vi "JSONRPC-BuildResponse.vi"(7 "ID":string="{\\\"jsonrpc\\\":\"2.0\",\\\"result\\\":%s,\\\"id\\\":%s}", 8 "error in":errorcluster, 11 "Result":string="{\\\"jsonrpc\\\":\"2.0\",\\\"result\\\":%s,\\\"id\\\":%s}") -> (0 "error out":errorcluster, 3 "JSONRPC Response":string)   [LabVIEW 2013]
doc: "Build a JSONRPC 2.0 response with <b>result</b>, or a JSONRPC 2.0 error response if <b>error in</b> contains an error. The response is bound to <b>ID</b>."
panel:
  # "BuildResponse"
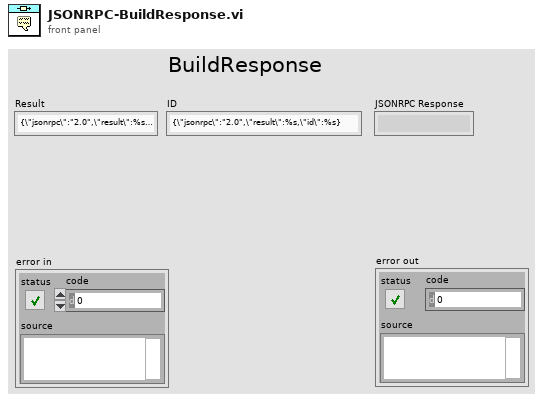
[diagram p1: front panel]
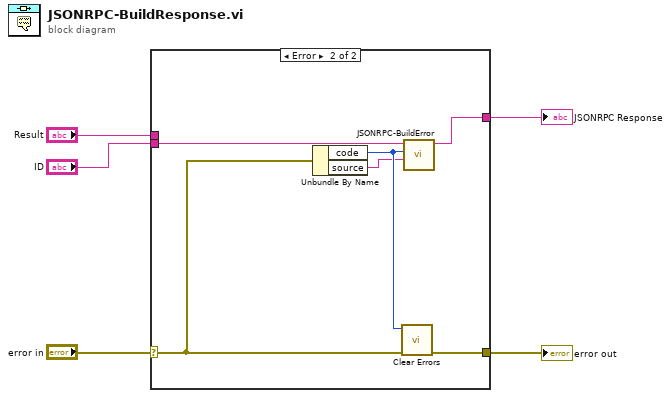
[diagram p0: block diagram]
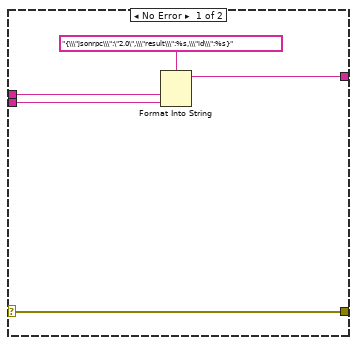
[diagram p2: hidden frame]
diagram:
  n1 = case shown="Error" "error in" {
    selector: "error in" -> [w7 w14]
    tunnel: "Result" -> [w9 _]
    tunnel: "ID" -> [w8 w16]
    tunnel: [w7 w13] -> w2
    tunnel: [w6 w15] -> w1
    frame No Error {
      n2 = Format Into String(format string="{\\\"jsonrpc\\\":\"2.0\",\\\"result\\\":%s,\\\"id\\\":%s}", w9, w8) -> (resulting string=w6:string)  [unwired: 2 in, 1 out]
    }
    frame Error {
      n3 = Unbundle By Name(w14) -> ("code"=w12:i32, "source"=w11:string)
      n4 = call <vilib>:"Clear Errors.vi"("error in (no error)"=w14, "specific error code to clear (0: all)"=w12) -> ("error out"=w13:errorcluster)  [unwired: 4 in, 1 out]
      n5 = call "JSONRPC-BuildError.vi"("Message"=w11, "Code"=w12, "ID"=w16) -> ("String"=w15:string)  [unwired: 8 in]
    }
  }
  "error out" <- w2
  "JSONRPC Response" <- w1
